vi "SetWebServicesURL.vi"(0 "reference in":refnum<class "VdTcpIP.lvclass">, 1 "WebServicesPostWebPage(*.asmx)":string, 2 "WebServicesURL_Location(http://...)":string, 5 "error in (no error)":errorcluster) -> (14 "reference out":refnum<class "VdTcpIP.lvclass">, 19 "error out":errorcluster)   [LabVIEW 2020, in "VdTcpIP.lvclass"]
uses:
  VdTcpIP.lvclass
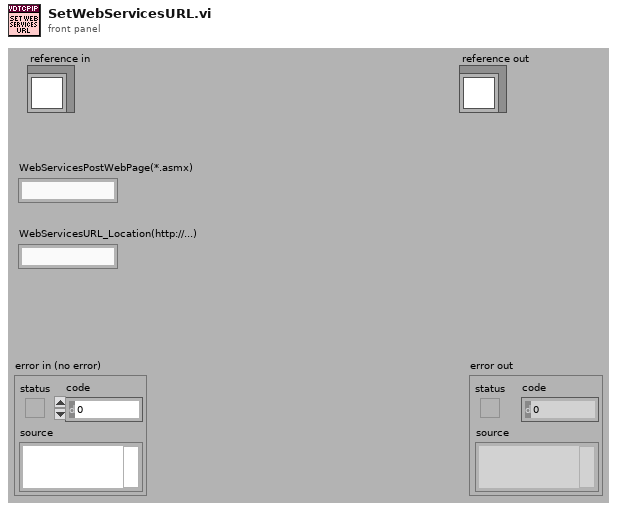
[diagram p1: front panel]
types:
  T1 = typedef "VdTcpIP.lvclass/ObjectAttributes.ctl" = cluster{"IP-Address":string, "Port":u16, "Connection":refnum<k5>, "Listener":refnum<k5>, "ListenerConnection":refnum<k5>, "Listner":bool, "ListnerProcessRunning":bool, "InConnections":refnum<k5>[], "InConnectionsIP":string[], "InConnectionAdded":refnum<notifier>, "RunVIOnNewConnection":variant, "DataToNewConnectionVI":cluster{"ControlName":string, "ControlValue":variant}[], "WebServicesURL_Location(http://...)":string, "WebServicesPostWebPage(*.asmx)":string, "Semaphore":T2, "AutoReConnectTimes":i32, "AutoReConnectInterval(ms)":i32, "ConnectionTimeout":i32}
  T2 = typedef "Semaphore RefNum" = refnum<k1>
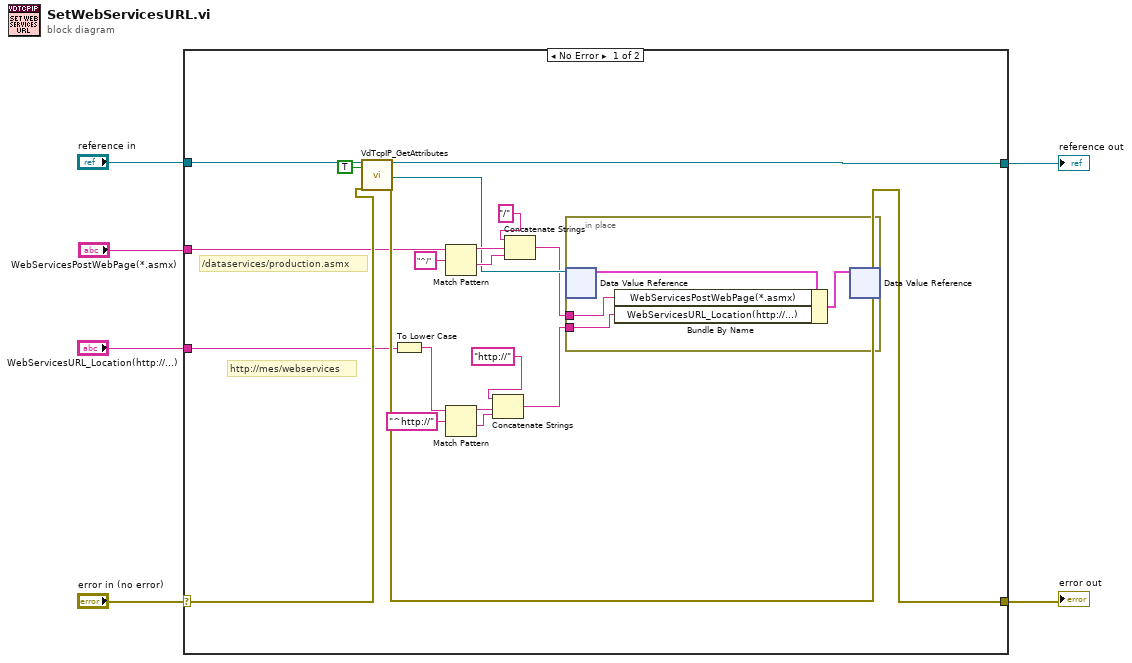
[diagram p0: block diagram]
diagram:
  n1 = case shown="No Error" "error in (no error)" {
    selector: "error in (no error)" -> [w23 w31]
    tunnel: [w25 w31] -> w5
    tunnel: [w22 w30] -> w3
    tunnel: "reference in" -> [w24 w30]
    tunnel: "WebServicesURL_Location(http://...)" -> [w15 _]
    tunnel: "WebServicesPostWebPage(*.asmx)" -> [w21 _]
    frame No Error {
      # "http://mes/webservices"
      # "/dataservices/production.asmx"
      n2 = call "VdTcpIP_GetAttributes.vi"("reference in"=w24, "OnlyGetDvrReference(False)"=TRUE, "error in (no error)"=w23) -> ("reference out"=w22:refnum<class "VdTcpIP.lvclass">, "DataRef"=w9:refnum<data-value>, "error out"=w25:errorcluster)  [unwired: 13 in, 1 out]
      n3 = To Lower Case(string=w15) -> (all lower case string=w11:string)
      n4 = Match Pattern(string=w21, regular expression="^/") -> (before substring=w19:string, after substring=w18:string)  [unwired: 3 out]
      n5 = Match Pattern(string=w11, regular expression="^http://") -> (before substring=w13:string, after substring=w12:string)  [unwired: 3 out]
      n6 = Concatenate Strings("http://" ("regular expression"), w13, w12) -> (w7:string)
      n7 = Concatenate Strings("/" ("regular expression"), w19, w18) -> (w8:string)
      n8 = in-place {
        in-place-border: w8 -> [w28]
        in-place-border: w7 -> [w27]
        n9 = in-place-dvr #1(w9) -> (w29:T1)  [unwired: 1 out]
        n10 = Bundle By Name(cluster=w29, "WebServicesPostWebPage(*.asmx)"=w28, "WebServicesURL_Location(http://...)"=w27) -> (w26:T1)
        n11 = in-place-dvr #1(w26) -> ()  [unwired: 2 out]
      }
    }
    frame Error {
    }
  }
  "error out" <- w5
  "reference out" <- w3
